vi "Drive Controller.vi"(8 "error in":errorcluster) -> ()   [LabVIEW 2017]
doc: "This VI executes continuously carrying out the current operation and responding to updates or new operation requests. It will often contain the timing or control code that is difficult to place directly in TeleOp. This VI generally opens all sensors and motors and isolates the rest of the robot code from knowing implementation details of how the operations are carried out."
uses:
  <vilib>/Rock Robotics/WPI/Framework/Completion Status.ctl
  Drive Setpoints.ctl
  Drive Operations.ctl
  Shared/RobotNeededPathData.ctl
  <vilib>/Rock Robotics/WPI/SafetyOutput/WPI_SafetyOutputConfigMenu.ctl
  <vilib>/Rock Robotics/SystemInterfaces/DIO/FPGA_DIOPWMChannel.ctl
  <vilib>/Rock Robotics/SystemInterfaces/DIO/FPGA_DIOChannel.ctl
  <vilib>/Rock Robotics/WPI/ThirdParty/Sensors/navX/_TypeDefs/FRIC_navX_DeviceNumbersTypeDef.ctl
  <vilib>/Rock Robotics/WPI/RobotDrive/WPI_RobotDriveOpen4MotorWithSPARK.vi
  <vilib>/Rock Robotics/WPI/Counter/WPI_CounterDigitalInputToDigitalSource.vi
  <vilib>/Rock Robotics/WPI/RobotDrive/WPI_RobotDriveOpen2MotorWithSPARK.vi
  <vilib>/addons/control/pid/pid.llb/PID (DBL).vi
  Drive Published Globals.vi
  <vilib>/addons/control/pid/NI_PID_pid.lvlib
  Configuration/Constants.vi
  Framework/Robot Global Data.vi
panel:
  in  "Integral Range":dbl=15.0
  out "PID Tuining":cluster{dbl, dbl}(graph)={170.0, 167.02}
  in  "Points":cluster{"X":dbl, "Y":dbl}[](array[cluster])=[{"X"=0.0, "Y"=0.0}, {"X"=0.01, "Y"=0.0}, {"X"=0.011, "Y"=0.17}, {"X"=1.0, "Y"=1.0}]
  in  "PID gains":T1={"proportional gain (Kc)"=0.01, "integral time (Ti, min)"=0.007, "derivative time (Td, min)"=0.0015} {"derivative time (Td, min)" format="%#_9g"}
  in  "Gains":T2={"FFV"=0.0059, "FFA"=0.0019, "Vel PID"={"P"=0.01, "I"=0.0, "D"=0.0}}
  in  "Interactive Values":T3={"Operation"=enum."Turn to Angle", "Left Speed"=-0.27, "Right Speed"=0.27, "Duration"=2.0, "Speed"=0.0, "Start Angle"=0.0, "Target Angle"=180.0, "Distance (inch)"=0.0, "Start Point (inch)"=0.0, "RobotNeededPathData"={"Path"=[], "MaxVel"=0.0, "MaxAccel"=-1.0, "Backwards?"=FALSE, "PointSpacing"=0.0, "LookaheadDist"=0.0, "Speed/Curve"=1.8, "SlowDistanceAtEnd"=12.0, "SlowSpeed"=15.0, "MaxDeAccel"=0.0}, "Start Point 2"=0.0} {"RobotNeededPathData"."SlowSpeed" format="%#_13g"; "RobotNeededPathData"."SlowDistanceAtEnd" format="%#_13g"; "RobotNeededPathData"."Speed/Curve" format="%#_13g"}
  in  "Buttons":cluster{"Execute Cmd":bool, "Abort Cmd":bool}
  out "Command Timing":cluster{"Start Time (ms)":u32, "Iterations":i32}={"Start Time (ms)"=372507, "Iterations"=0}
  out "Status":T6
  out "Setpoints":T7(graph)
  out "Current\nCmd":string="Started at  14:51:47.884\nDefault: Reserve,  L 0.0, R 0.0, D 0.000000"
  # "Tip: The graph shows the motor setpoints. It may also be helpful to observe inputs and sensor values.\nYou may also want to display tuning or debugging controls."
  # ".0088"
  # ".0017"
  # ".02"
  # "Interactive Command: You may fill in the settings for a command\nand schedule it with the Execute button. You can observe and abort\nany command while fine tuning the code for the controller."
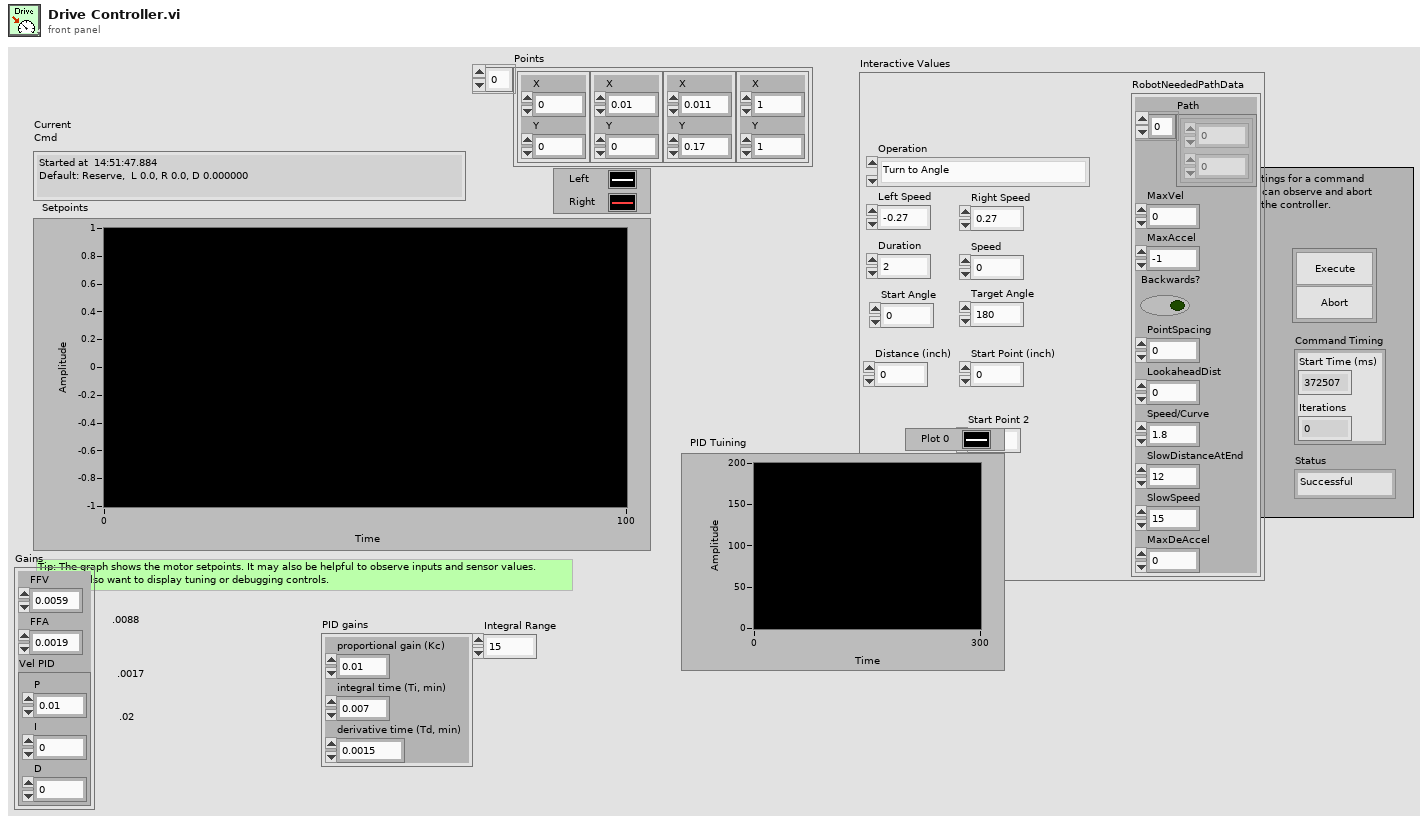
[diagram p1: front panel]
types:
  T1 = cluster{"proportional gain (Kc)":dbl, "integral time (Ti, min)":dbl, "derivative time (Td, min)":dbl}
  T2 = cluster{"FFV":dbl, "FFA":dbl, "Vel PID":cluster{"P":dbl, "I":dbl, "D":dbl}}
  T3 = typedef "Drive Setpoints.ctl" = cluster{"Operation":T4, "Left Speed":dbl, "Right Speed":dbl, "Duration":dbl, "Speed":dbl, "Start Angle":dbl, "Target Angle":dbl, "Distance (inch)":dbl, "Start Point (inch)":dbl, "RobotNeededPathData":T5, "Start Point 2":dbl}
  T4 = typedef "Drive Operations.ctl" = enum16{"Reserve", "Read Current", "Immediate", "Drive for Time", "Drive for Distance", "Turn to Angle", "Arc Turn", "Drive Path", "Drive To Cube"}
  T5 = typedef "RobotNeededPathData.ctl" = cluster{"Path":cluster{dbl, dbl}[], "MaxVel":dbl, "MaxAccel":dbl, "Backwards?":bool, "PointSpacing":dbl, "LookaheadDist":dbl, "Speed/Curve":dbl, "SlowDistanceAtEnd":dbl, "SlowSpeed":dbl, "MaxDeAccel":dbl}
  T6 = typedef "Completion Status.ctl" = enum16{"Successful", "Aborted", "Incomplete"}
  T7 = cluster{"Left Setpoint":dbl, "Right Setpoint":dbl}
  T8 = typedef "FPGA_DIOChannel.ctl" = enum8{"DIO 0", "DIO 1", "DIO 2", "DIO 3", "DIO 4", "DIO 5", "DIO 6", "DIO 7", "DIO 8", "DIO 9", "DIO MXP 0", "DIO MXP 1", "DIO MXP 2", "DIO MXP 3", "DIO MXP 4", "DIO MXP 5", "DIO MXP 6", "DIO MXP 7", "DIO MXP 8", "DIO MXP 9", "DIO MXP 10", "DIO MXP 11", "DIO MXP 12", "DIO MXP 13", "DIO MXP 14", "DIO MXP 15", "SPI Port CS1", "SPI Port CS2", "SPI Port CS3", "SPI Port MISO", "SPI Port MOSI", "Invalid"}
  T9 = typedef "FPGA_DIOPWMChannel.ctl" = enum8{"PWM 0", "PWM 1", "PWM 2", "PWM 3", "PWM 4", "PWM 5", "PWM 6", "PWM 7", "PWM 8", "PWM 9", "PWM MXP 0", "PWM MXP 1", "PWM MXP 2", "PWM MXP 3", "PWM MXP 4", "PWM MXP 5", "PWM MXP 6", "PWM MXP 7", "PWM MXP 8", "PWM MXP 9", "Invalid"}
  T10 = typedef "WPI_SafetyOutputConfigMenu.ctl" = enum16{"Enable", "Disable"}
  T11 = typedef "WPI_DigitalInputDevRef.ctl" = cluster{"DevStatus":errorcluster, "DIO Channel":T8}
  T12 = typedef "FPGA_CounterEncoderSourceConvertionLVSourceType.ctl" = cluster{"DevStatus":errorcluster, "AnalogTriggerMode?":bool, "DigitalMode":cluster{"DIO Channel":T13}, "AnalogTriggerMode":cluster{"AnalogTriggerIndex":T14, "OutputType":T15}}
  T13 = typedef "FPGA_DIODigitalSourceChannel.ctl" = enum8{"DIO 0", "DIO 1", "DIO 2", "DIO 3", "DIO 4", "DIO 5", "DIO 6", "DIO 7", "DIO 8", "DIO 9", "DIO MXP 0", "DIO MXP 1", "DIO MXP 2", "DIO MXP 3", "DIO MXP 4", "DIO MXP 5", "DIO MXP 6", "DIO MXP 7", "DIO MXP 8", "DIO MXP 9", "DIO MXP 10", "DIO MXP 11", "DIO MXP 12", "DIO MXP 13", "DIO MXP 14", "DIO MXP 15", "Disabled"}
  T14 = typedef "FPGA_AnalogTriggerIndex.ctl" = enum8{"Trig 0", "Trig 1", "Trig 2", "Trig 3", "Trig 4", "Trig 5", "Trig 6", "Trig 7", "Invalid"}
  T15 = typedef "FPGA_AnalogTriggerOutType.ctl" = enum16{"InWindow", "TriggerState", "Rising", "Falling"}
  T16 = typedef "WPI_RobotDriveDevRef.ctl" = cluster{"DevStatus":errorcluster, "Motors[]":T17[], "Square Inputs":bool, "Max Output":dbl}
  T17 = typedef "WPI_MotorControlDeviceRef.ctl" = cluster{"DeviceStatus":errorcluster, "Type":T18, "PWM":cluster{"PWM Channel":T9, "DeadBand":T19}, "CAN":cluster{"Device Number":u8, "SetOutput VI Ref":variant, "GetOutput VI Ref":variant, "Enable VI Ref":variant, "Disable VI Ref":variant, "Data":variant}, "Invert":bool, "DIO PWM":cluster{"PWM \"Enable\" Channel":T9, "DIOChannel":T8, "PWM Rate":dbl}}
  T18 = typedef "WPI_MotorControlType.ctl" = enum16{"PWM", "CAN", "DIO PWM"}
  T19 = typedef "WPI_PWMDeadband.ctl" = cluster{"Name":string, "maxPositivePwm":i32, "minPositivePwm":i32, "centerPwm":i32, "maxNegativePwm":i32, "minNegativePwm":i32, "angularRange":u16}
  T20 = typedef "WPI_EncoderDevRef.ctl" = cluster{"DevStatus":errorcluster, "EncoderIndex":T21, "CounterIndex":T22, "DistancePerCount":dbl, "Decoding Type":T23}
  T21 = typedef "FPGA_EncoderIdx.ctl" = enum8{"Enc 0", "Enc 1", "Enc 2", "Enc 3", "Enc 4", "Enc 5", "Enc 6", "Enc 7", "Invalid"}
  T22 = typedef "FPGA_CounterCtrSystemIndex.ctl" = enum8{"Ctr 0", "Ctr 1", "Ctr 2", "Ctr 3", "Ctr 4", "Ctr 5", "Ctr 6", "Ctr 7", "Invalid"}
  T23 = typedef "WPI_EncoderType.ctl" = enum16{"1x", "2x", "4x"}
  T24 = typedef "Command Status Info.ctl" = cluster{"Name":string, "Status":T6, "notifier out":T25}
  T25 = typedef "Completion Notifier.ctl" = refnum<notifier>
  T26 = cluster{"SubSystem Data":T3, cluster{"Start Time (ms)":u32, "Iterations":i32}, cluster{"Command Info":T24, "Description":string, "Default Command":T3, "queue out":refnum<queue>, "Subsystem Name":string}}
  T27 = typedef "FRIC_navX_DeviceNumbersTypeDef.ctl" = enum16{"Dev0", "Dev1", "Dev2", "Dev3"}
  T28 = cluster{"dx/dt":dbl, "dx/dt":dbl, "Yaw":dbl, cluster{dbl, dbl}}
  T29 = cluster{"LeftDistance":dbl, "RightDistance":dbl, "LeftVelocity":dbl, "RightVelocity":dbl, "Angle":dbl, "Location":cluster{dbl, dbl}}
  T30 = cluster{"Yaw":dbl, "Roll":dbl, "Pitch":dbl, "Heading":dbl, "Fused Heading":dbl}
  T31 = cluster{"SubSystem Data":T3, cluster{"Start Time (ms)":u32, "Iterations":i32}, "Default Command Arguments":cluster{"Command Info":T24, "Description":string, "Default Command":T3, "queue out":refnum<queue>, "Subsystem Name":string}}
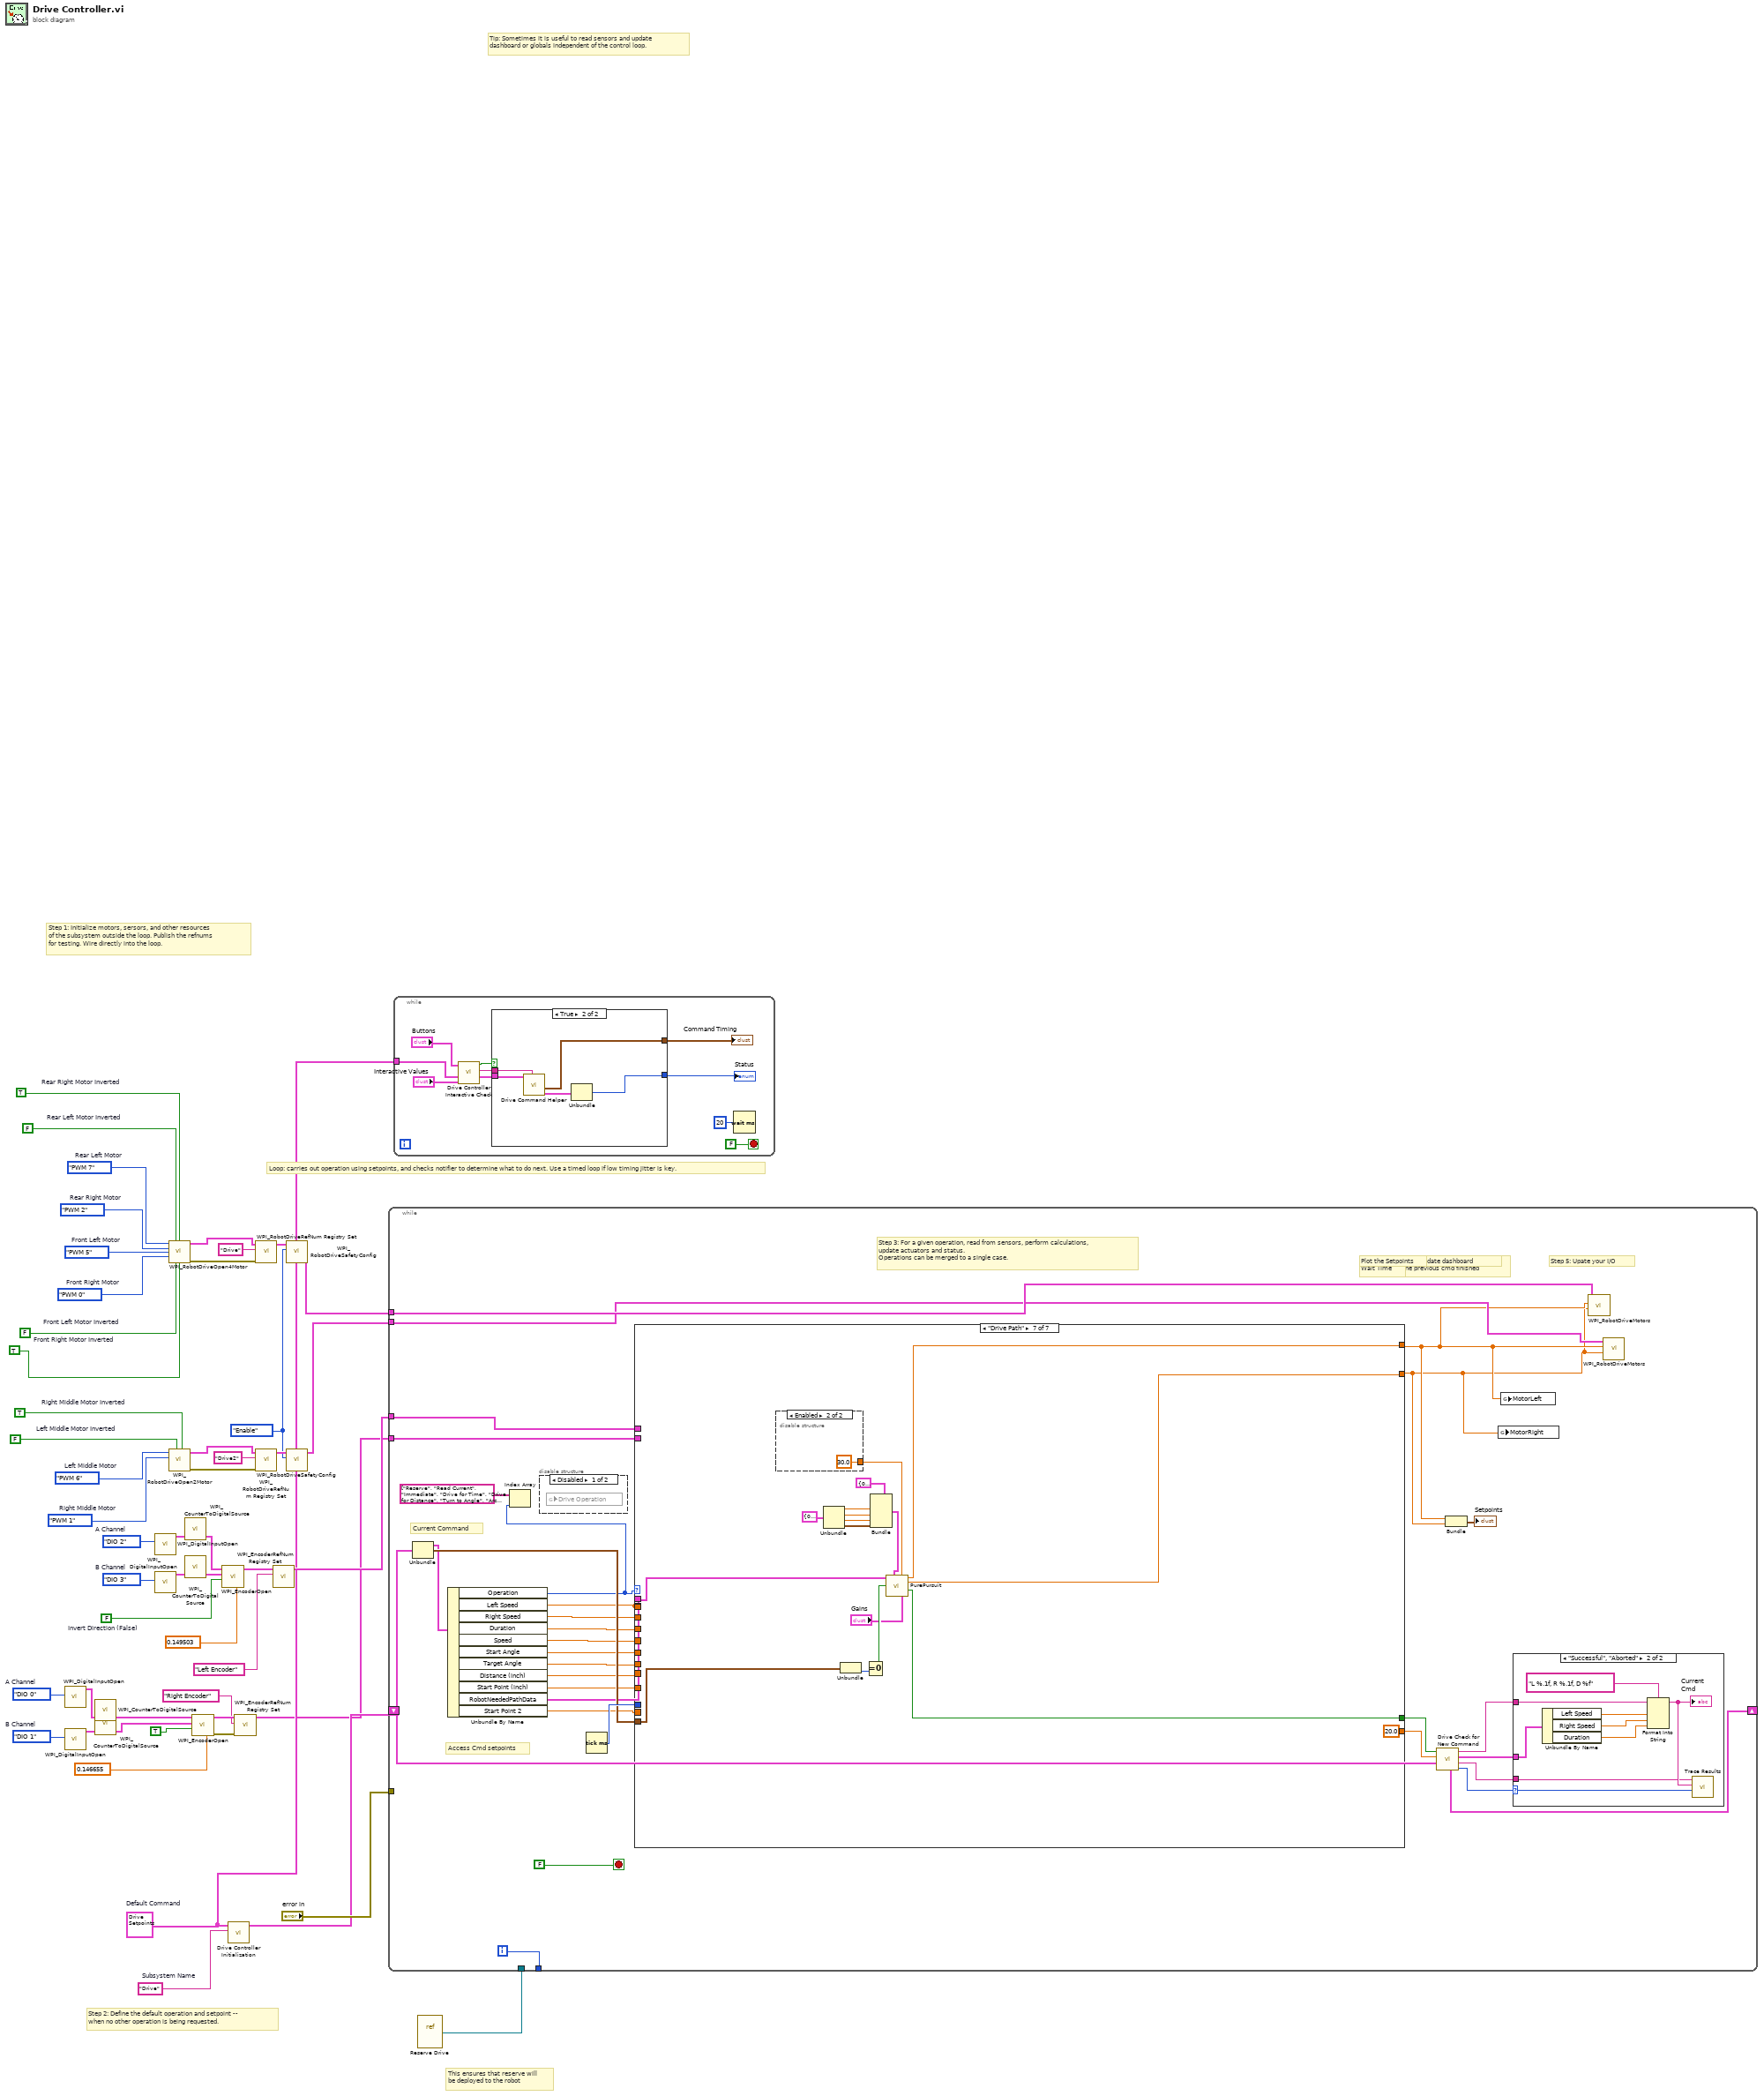
[diagram p0: block diagram]
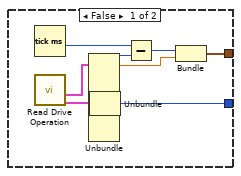
[diagram p2: hidden frame]
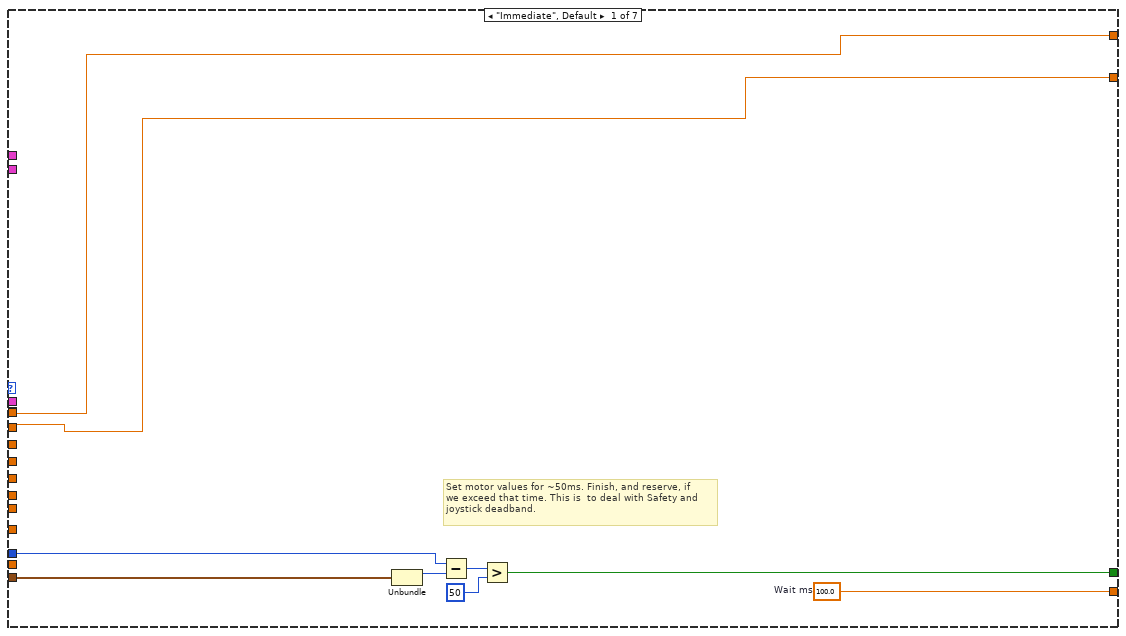
[diagram p4: hidden frame]
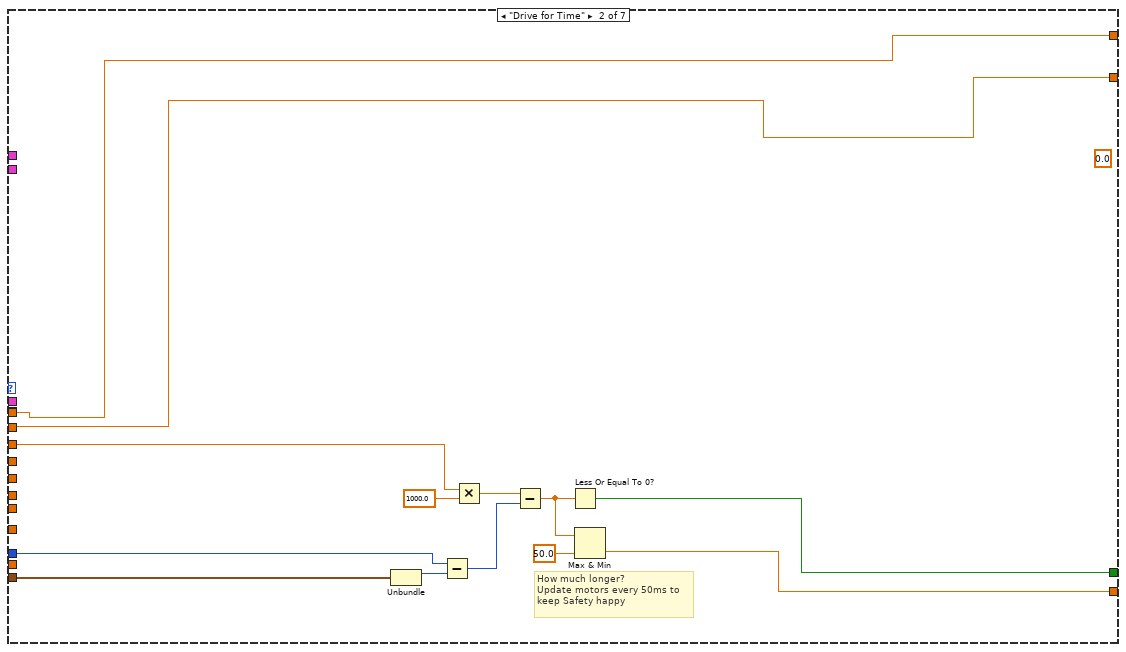
[diagram p5: hidden frame]
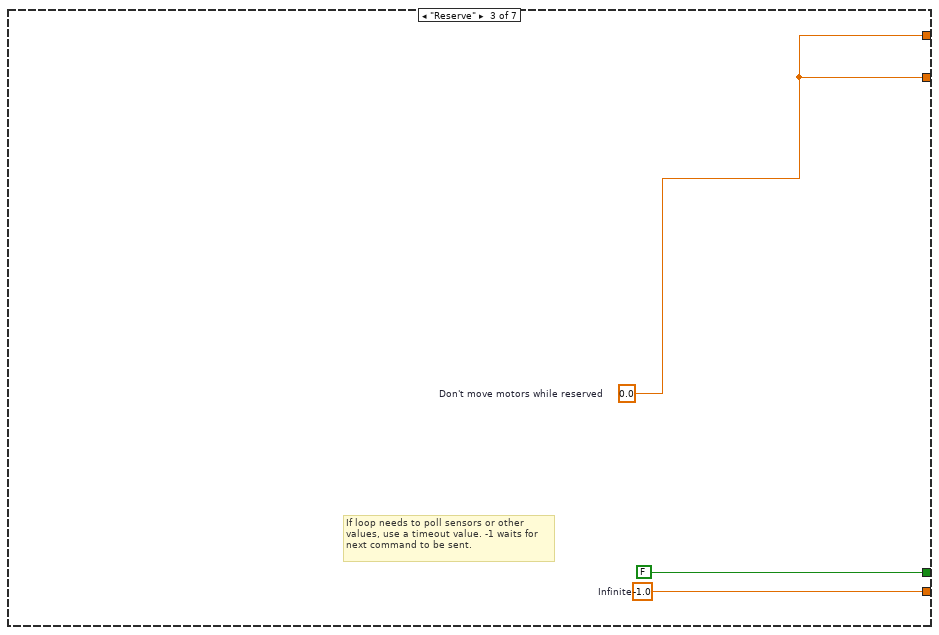
[diagram p6: hidden frame]
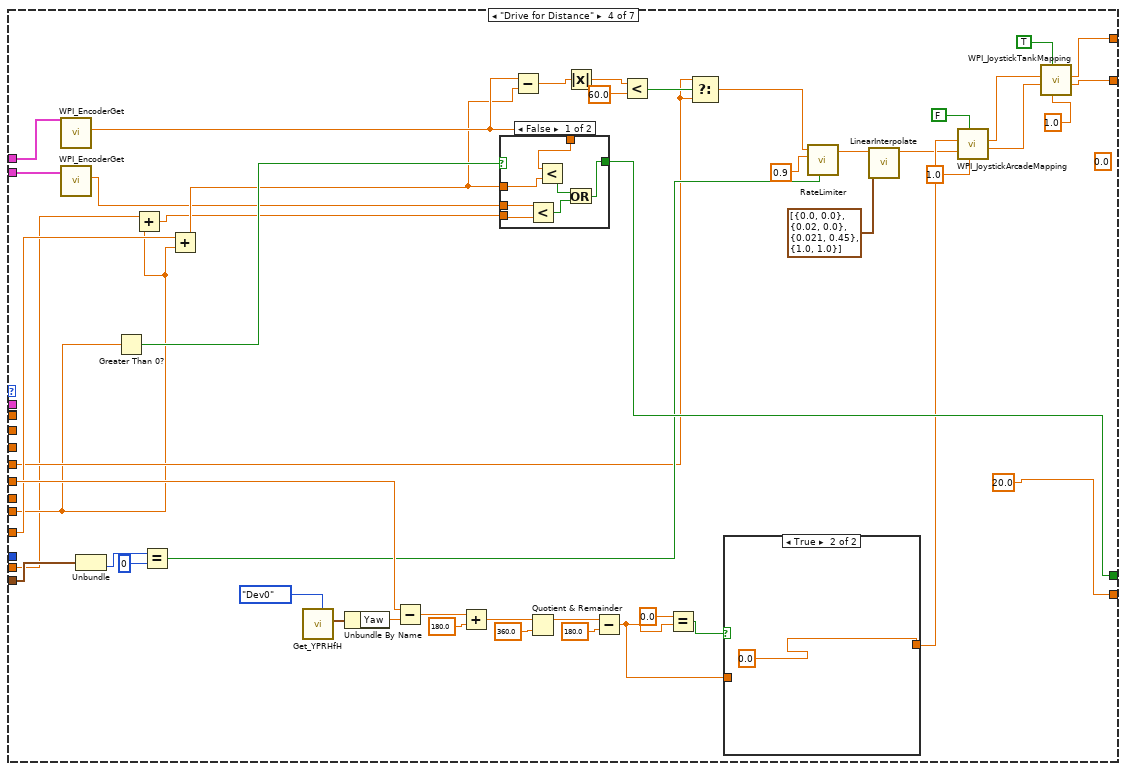
[diagram p7: hidden frame]
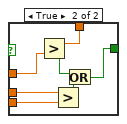
[diagram p8: hidden frame]
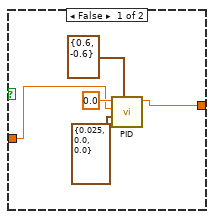
[diagram p9: hidden frame]
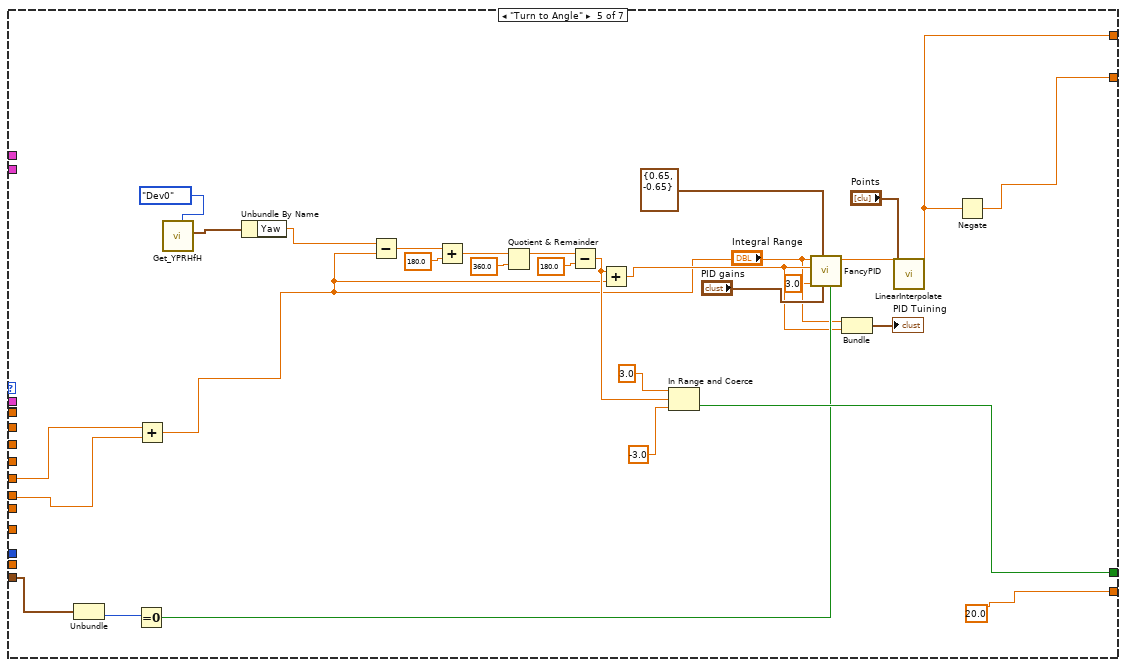
[diagram p10: hidden frame]
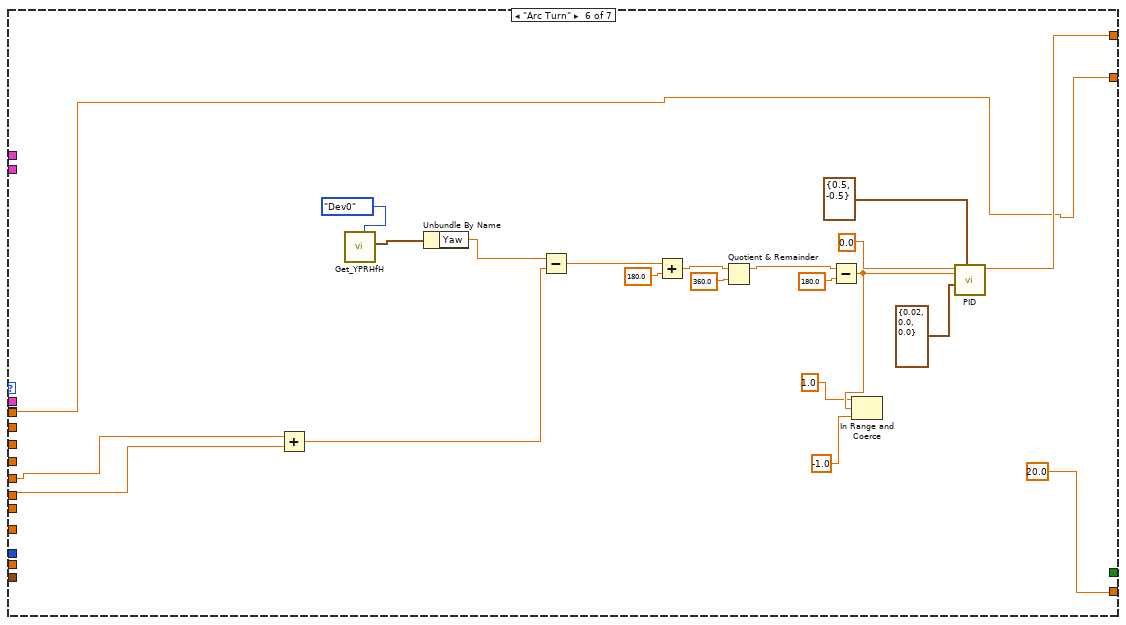
[diagram p11: hidden frame]
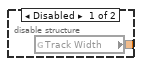
[diagram p12: hidden frame]
diagram:
  w4 = FPGA_DIOChannel."DIO 1"  # B Channel
  w7 = FPGA_DIOChannel."DIO 0"  # A Channel
  w13 = T3 {"Operation"=enum."Reserve", "Left Speed"=0.0, "Right Speed"=0.0, "Duration"=0.0, "Speed"=0.0, "Start Angle"=0.0, "Target Angle"=0.0, "Distance (inch)"=0.0, "Start Point (inch)"=0.0, "RobotNeededPathData"={"Path"=[], "MaxVel"=0.0, "MaxAccel"=0.0, "Backwards?"=FALSE, "PointSpacing"=0.0, "LookaheadDist"=0.0, "Speed/Curve"=1.8, "SlowDistanceAtEnd"=12.0, "SlowSpeed"=15.0, "MaxDeAccel"=0.0}, "Start Point 2"=0.0}  # Default Command
  w20 = TRUE  # Right Middle Motor Inverted
  w21 = FALSE  # Left Middle Motor Inverted
  w24 = FPGA_DIOPWMChannel."PWM 1"  # Right Middle Motor
  w25 = FPGA_DIOPWMChannel."PWM 6"  # Left Middle Motor
  w34 = FALSE  # Invert Direction (False)
  w27 = FPGA_DIOChannel."DIO 3"  # B Channel
  w28 = FPGA_DIOChannel."DIO 2"  # A Channel
  w36 = TRUE  # Front Right Motor Inverted
  w37 = FALSE  # Front Left Motor Inverted
  w38 = TRUE  # Rear Right Motor Inverted
  w39 = FALSE  # Rear Left Motor Inverted
  w40 = FPGA_DIOPWMChannel."PWM 0"  # Front Right Motor
  w41 = FPGA_DIOPWMChannel."PWM 5"  # Front Left Motor
  w42 = FPGA_DIOPWMChannel."PWM 2"  # Rear Right Motor
  w43 = FPGA_DIOPWMChannel."PWM 7"  # Rear Left Motor
  w15 = WPI_SafetyOutputConfigMenu."Enable" ("mode")
  w51 = "Drive"  # Subsystem Name
  # "Step 1: Initialize motors, sersors, and other resources\nof the subsystem outside the loop. Publish the refnums\nfor testing. Wire directly into the loop."
  # "Step 2: Define the default operation and setpoint --\nwhen no other operation is being requested."
  # "This ensures that reserve will\nbe deployed to the robot"
  # "Tip: Sometimes it is useful to read sensors and update\ndashboard or globals independent of the control loop."
  # "Loop: carries out operation using setpoints, and checks notifier to determine what to do next. Use a timed loop if low timing jitter is key."
  n1 = call <vilib>:"WPI_DigitalInputOpen.vi"("DIO Channel"=w7) -> ("DigitalInputDevRef"=w8:T11)  [unwired: 1 in, 9 out]
  n2 = call <vilib>:"WPI_DigitalInputOpen.vi"("DIO Channel"=w4) -> ("DigitalInputDevRef"=w5:T11)  [unwired: 1 in, 9 out]
  n3 = call-poly <vilib>:"WPI_CounterToDigitalSource.vi"("DigitalInputDevRef"=w8) -> ("Digital Source"=w9:T12)  [unwired: 6 out]
  n4 = call-poly <vilib>:"WPI_CounterToDigitalSource.vi"("DigitalInputDevRef"=w5) -> ("Digital Source"=w6:T12)  [unwired: 6 out]
  n5 = call <vilib>:"WPI_DigitalInputOpen.vi"("DIO Channel"=w28) -> ("DigitalInputDevRef"=w31:T11)  [unwired: 1 in, 9 out]
  n6 = call <vilib>:"WPI_DigitalInputOpen.vi"("DIO Channel"=w27) -> ("DigitalInputDevRef"=w30:T11)  [unwired: 1 in, 9 out]
  n7 = call-poly <vilib>:"WPI_RobotDriveOpen4Motor.vi"("Rear Left Motor"=w43, "Rear Left Motor Inverted"=w39, "Rear Right Motor Inverted"=w38, "Rear Right Motor"=w42, "Front Left Motor"=w41, "Front Right Motor"=w40, "Front Left Motor Inverted"=w37, "Front Right Motor Inverted"=w36) -> ("RobotDriveDevRef"=w50:T16, "error out"=w48:errorcluster)  [unwired: 6 in]
  n8 = call-poly <vilib>:"WPI_RobotDriveOpen2Motor.vi"("Right Motor Inverted"=w20, "Left Motor Inverted"=w21, "Right Motor"=w24, "Left Motor"=w25) -> ("error out"=w19:errorcluster, "RobotDriveDevRef"=w23:T16)  [unwired: 6 in]
  n9 = call-poly <vilib>:"WPI_CounterToDigitalSource.vi"("DigitalInputDevRef"=w31) -> ("Digital Source"=w32:T12)  [unwired: 6 out]
  n10 = call-poly <vilib>:"WPI_CounterToDigitalSource.vi"("DigitalInputDevRef"=w30) -> ("Digital Source"=w29:T12)  [unwired: 6 out]
  n11 = call <vilib>:"WPI_EncoderOpen.vi"("DistancePerCount"=0.146655, "Invert Direction (False)"=TRUE, "BSource"=w6, "ASource"=w9) -> ("error out"=w11:errorcluster, "EncoderDevRef"=w10:T20)  [unwired: 4 in, 2 out]
  n12 = call <vilib>:"WPI_EncoderOpen.vi"("DistancePerCount"=0.149503, "Invert Direction (False)"=w34, "BSource"=w29, "ASource"=w32) -> ("EncoderDevRef"=w33:T20)  [unwired: 4 in, 3 out]
  n13 = call "Drive Controller Initialization.vi"("Subsystem Name"=w51, "Default Command"=w13) -> ("Current Command"=w45:T26)  [unwired: 9 in]
  n14 = call <vilib>:"WPI_EncoderRefNum Registry Set.vi"("error in (no error)"=w11, "refnum name"="Right Encoder", "EncoderDevRef"=w10) -> ("EncoderDevRef"=w12:T20)  [unwired: 7 in, 1 out]
  n15 = call <vilib>:"WPI_RobotDriveRefNum Registry Set.vi"("error in (no error)"=w48, "refnum name"="Drive", "RobotDriveDevRef"=w50) -> ("RobotDriveDevRef"=w18:T16)  [unwired: 1 in, 7 out]
  n16 = call <vilib>:"WPI_RobotDriveRefNum Registry Set.vi"("error in (no error)"=w19, "refnum name"="Drive2", "RobotDriveDevRef"=w23) -> ("RobotDriveDevRef"=w17:T16)  [unwired: 7 in, 1 out]
  n17 = call <vilib>:"WPI_EncoderRefNum Registry Set.vi"("refnum name"="Left Encoder", "EncoderDevRef"=w33) -> ("EncoderDevRef"=w26:T20)  [unwired: 8 in, 1 out]
  n18 = call <vilib>:"WPI_RobotDriveSafetyConfig.vi"("mode"=w15, "RobotDriveDevRef"=w18) -> ("RobotDriveDevRef"=w47:T16)  [unwired: 8 in, 1 out]
  n19 = call <vilib>:"WPI_RobotDriveSafetyConfig.vi"("mode"=w15, "RobotDriveDevRef"=w17) -> ("RobotDriveDevRef"=w16:T16)  [unwired: 8 in, 1 out]
  n20 = while {
    tunnel: w13 -> [w53]
    stop <- FALSE stop-if-true
    n21 = call "Drive Controller Interactive Check.vi"("Interactive Command In"="Interactive Values", "Default Command"=w53, "Buttons"="Buttons") -> ("Interactive Command Out"=w55:T3, "Trace String"=w56:string, "Schedule"=w57:bool)  [unwired: 6 in]
    n22 = case shown="True" w57 {
      tunnel: [w66 w74] -> w58
      tunnel: [w65 w70] -> w59
      tunnel: w56 -> [_ w72]
      tunnel: w55 -> [_ w71]
      frame False {
        n23 = Tick Count (ms)() -> (millisecond timer value=w69:u32)
        n24 = call "Read Drive Operation.vi"() -> ("Command Info"=w63:T24, "SubSystem Data"=w62:T3)  [unwired: 9 in, 1 out]
        n25 = Unbundle(w62) -> ("Operation"=w67:T4, "Left Speed"=w64:dbl)  [unwired: 9 out]
        n26 = Unbundle(w63) -> ("Status"=w66:T6)  [unwired: 2 out]
        n27 = Subtract(x=w69, y=w67) -> (x-y=w68:u32)
        n28 = Bundle(w68, "Left Speed"=w64) -> (w65:cluster{u32, "Left Speed":dbl})  [unwired: 1 in]
      }
      frame True {
        n29 = call "Drive Command Helper.vi"("Description"=w72, "SubSystem Data"=w71) -> ("Command Info Out"=w73:T24, "Command Timing"=w70:cluster{"Start Time (ms)":u32, "Iterations":i32})  [unwired: 7 in, 1 out]
        n30 = Unbundle(w73) -> ("Status"=w74:T6)  [unwired: 2 out]
      }
    }
    "Status" <- w58
    "Command Timing" <- w59
    n31 = Wait (ms)(milliseconds to wait=u32 20) -> ()  [unwired: 1 out]
  }
  n32 = vi-ref "Reserve Drive.vi"() -> (w44:refnum<vi>)
  n33 = while {
    shift-right: [w102] -> _
    shift-left: w45 -> [w75]
    tunnel: [w105] -> _
    tunnel: w47 -> [w84]
    tunnel: "error in" -> [_]
    tunnel: w44 -> [_]
    tunnel: w26 -> [w82]
    tunnel: w16 -> [w83]
    tunnel: w12 -> [w81]
    i -> [w105]
    stop <- FALSE stop-if-true
    # "Plot the Setpoints"
    # "Step 5: Upate your I/O"
    # "Step 4: Format a string to describe this\ncmd and how the previous cmd finished"
    # "Current Command"
    # "Update motors and update dashboard"
    # "Access Cmd setpoints"
    # "Finished? &\nWait Time"
    # "Step 3: For a given operation, read from sensors, perform calculations,\nupdate actuators and status.\nOperations can be merged to a single case."
    n34 = Unbundle(w75) -> ("SubSystem Data"=w85:T3, w96:cluster{"Start Time (ms)":u32, "Iterations":i32})  [unwired: 1 out]
    n35 = Unbundle By Name(w85) -> ("Operation"=w77:T4, "Left Speed"=w94:dbl, "Right Speed"=w93:dbl, "Duration"=w92:dbl, "Speed"=w91:dbl, "Start Angle"=w90:dbl, "Target Angle"=w89:dbl, "Distance (inch)"=w88:dbl, "Start Point (inch)"=w87:dbl, "RobotNeededPathData"=w86:T5, "Start Point 2"=w80:dbl)
    n36 = Index Array(array=string[] ["Reserve", "Read Current", "Immediate", "Drive for Time", "Drive for Distance", "Turn to Angle", "Arc Turn", "Drive Path", "Drive To Cube"] ("Strings []"), index=w77) -> ()  [unwired: 1 out]
    n37 = disable-structure shown="Disabled" {
      frame Disabled {
        n38 = global read "Robot Global Data.vi" "Drive Operation"() -> ()  [unwired: 1 in]
      }
      frame Enabled {
      }
    }
    n39 = Tick Count (ms)() -> (millisecond timer value=w104:u32)
    n40 = case shown="\"Drive Path\"" w77 {
      tunnel: [w115 w119 w131 20.0 ("Infinite") 20.0 ("Infinite") 20.0 ("Infinite") 20.0 ("Infinite")] -> w101
      tunnel: [w110 w123 FALSE ("ignore previous (F)") w167 w222 _ w264] -> w100
      tunnel: w96 -> [w109 w125 _ w148 w212 _ w263]
      tunnel: w104 -> [w111 w122 _ _ _ _ _]
      tunnel: [w108 w117 w129 w153 w210 w231 w266] -> w79
      tunnel: [w107 w116 w129 w154 w209 w230 w265] -> w78
      tunnel: w91 -> [_ _ _ w137 _ _ _]
      tunnel: w88 -> [_ _ _ w135 _ _ _]
      tunnel: w92 -> [_ w118 _ _ _ _ _]
      tunnel: w94 -> [w108 _ _ _ _ w230 _]
      tunnel: w93 -> [w107 w116 _ _ _ _ _]
      tunnel: w82 -> [_ _ _ w165 _ _ _]
      tunnel: w90 -> [_ _ _ w161 w225 w234 _]
      tunnel: w89 -> [_ _ _ _ w224 w233 _]
      tunnel: w87 -> [_ _ _ w160 _ _ _]
      tunnel: w94 -> [_ w117 _ _ _ _ _]
      tunnel: w86 -> [_ _ _ _ _ _ w267]
      tunnel: w81 -> [_ _ _ w136 _ _ _]
      tunnel: w80 -> [_ _ _ w134 _ _ _]
      frame "Immediate", Default {
        w115 = 100.0  # Wait ms
        # "Set motor values for ~50ms. Finish, and reserve, if\nwe exceed that time. This is  to deal with Safety and\njoystick deadband."
        n41 = Unbundle(w109) -> ("Start Time (ms)"=w112:u32)  [unwired: 1 out]
        n42 = Subtract(x=w111, y=w112) -> (x-y=w113:u32)
        n43 = Greater?(x=w113, y=u8 50 ("Left Motor")) -> (0:w110:bool)
      }
      frame "Drive for Time" {
        (unwired) 0.0 ("output")
        # "How much longer?\nUpdate motors every 50ms to\nkeep Safety happy"
        n44 = Unbundle(w125) -> ("Start Time (ms)"=w124:u32)  [unwired: 1 out]
        n45 = Subtract(x=w122, y=w124) -> (x-y=w128:u32)
        n46 = Multiply(x=w118, y=1000.0) -> (x*y=w127:dbl)
        n47 = Subtract(x=w127, y=w128) -> (x-y=w121:dbl)
        n48 = Less Or Equal To 0?(x=w121) -> (x <= 0?=w123:bool)
        n49 = Max & Min(x=w121, y=50.0) -> (min(x,y)=w119:dbl)  [unwired: 1 out]
      }
      frame "Reserve" {
        w129 = 0.0  # Don't move motors while reserved
        w131 = -1.0  # Infinite
        # "If loop needs to poll sensors or other\nvalues, use a timeout value. -1 waits for\nnext command to be sent."
      }
      frame "Drive for Distance" {
        (unwired) 0.0 ("output")
        n50 = call <vilib>:"WPI_EncoderGet.vi"("EncoderDevRef"=w165) -> ("Distance"=w144:dbl)  [unwired: 5 in, 5 out]
        n51 = call <vilib>:"WPI_EncoderGet.vi"("EncoderDevRef"=w136) -> ("Distance"=w132:dbl)  [unwired: 5 in, 5 out]
        n52 = Unbundle(w148) -> ("Iterations"=w147:i32)  [unwired: 1 out]
        n53 = Greater Than 0?(x=w135) -> (x > 0?=w159:bool)
        n54 = Add(x=w134, y=w135) -> (x+y=w133:dbl)
        n55 = Equal?(x=w147, y=0) -> (x = y?=w145:bool)
        n56 = Add(x=w160, y=w135) -> (x+y=w143:dbl)
        n57 = call <vilib>:"Get_YPRHfH.vi"("Device Number"=FRIC_navX_DeviceNumbersTypeDef."Dev0") -> ("YRPHfH"=w179:T30)  [unwired: 10 in]
        n58 = Unbundle By Name(w179) -> ("Yaw"=w170:dbl)
        n59 = Subtract(x=w161, y=w170) -> (x-y=w169:dbl)
        n60 = Add(x=w169, y=180.0) -> (x+y=w174:dbl)
        n61 = case shown="False" w159 {
          tunnel: w144 -> [w185 w193]
          tunnel: w143 -> [w186 w192]
          tunnel: [w183 w187] -> w167
          tunnel: w133 -> [w181 w191]
          tunnel: w132 -> [w182 w190]
          frame False {
            n62 = Less?(x=w182, y=w181) -> (x < y?=w180:bool)
            n63 = Less?(x=w185, y=w186) -> (x < y?=w184:bool)
            n64 = Or(x=w184, y=w180) -> (x .or. y?=w183:bool)
          }
          frame True {
            n65 = Greater?(x=w193, y=w192) -> (0:w189:bool)
            n66 = Greater?(x=w190, y=w191) -> (0:w188:bool)
            n67 = Or(x=w189, y=w188) -> (x .or. y?=w187:bool)
          }
        }
        n68 = Subtract(x=w144, y=w143) -> (x-y=w142:dbl)
        n69 = Quotient & Remainder(x=w174, y=360.0) -> (x-y*floor(x/y)=w172:dbl)  [unwired: 1 out]
        n70 = Absolute Value(x=w142) -> (abs(x)=w141:dbl)
        n71 = Subtract(x=w172, y=180.0) -> (x-y=w168:dbl)
        n72 = Less?(x=w141, y=60.0) -> (x < y?=w139:bool)
        n73 = Equal?(x=0.0, y=w168) -> (x = y?=w177:bool)
        n74 = Select(t=w137, s=w139, f=w137) -> (s? t:f=w138:dbl)
        n75 = case shown="True" w177 {
          tunnel: [w194 0.0] -> w162
          tunnel: w168 -> [w195 _]
          frame False {
            n76 = call-poly <vilib>:"PID.vi"("output range"=cluster{"output high":dbl, "output low":dbl} {"output high"=0.6, "output low"=-0.6}, "PID gains"=T1 {"proportional gain (Kc)"=0.025, "integral time (Ti, min)"=0.0, "derivative time (Td, min)"=0.0}, "process variable"=w195, "setpoint"=0.0) -> ("output"=w194:dbl)  [unwired: 6 in, 1 out]
          }
          frame True {
          }
        }
        n77 = call "RateLimiter.vi"("Reset"=w145, "Max dx/dt"=0.9, "Input"=w138) -> ("Output"=w156:dbl)  [unwired: 8 in]
        n78 = call "LinearInterpolate.vi"("Points"=cluster{"X":dbl, "Y":dbl}[] [{"X"=0.0, "Y"=0.0}, {"X"=0.02, "Y"=0.0}, {"X"=0.021, "Y"=0.45}, {"X"=1.0, "Y"=1.0}], "Value"=w156) -> ("Output"=w157:dbl)  [unwired: 9 in]
        n79 = call <vilib>:"WPI_JoystickArcadeMapping.vi"("Max Output"=1.0, "Square Inputs"=FALSE, "Y axis value"=w157, "X axis value"=w162) -> ("Right Motor Value"=w152:dbl, "Left Motor Value"=w151:dbl)  [unwired: 6 in]
        n80 = call <vilib>:"WPI_JoystickTankMapping.vi"("Max Output"=1.0, "Square Inputs"=TRUE, "Right axis value"=w152, "Left axis value"=w151) -> ("Right Motor Value"=w154:dbl, "Left Motor Value"=w153:dbl)  [unwired: 6 in]
      }
      frame "Turn to Angle" {
        n81 = Unbundle(w212) -> ("Iterations"=w211:i32)  [unwired: 1 out]
        n82 = Equal To 0?(x=w211) -> (x = 0?=w205:bool)
        n83 = Add(x=w225, y=w224) -> (x+y=w202:dbl)
        n84 = call <vilib>:"Get_YPRHfH.vi"("Device Number"=FRIC_navX_DeviceNumbersTypeDef."Dev0") -> ("YRPHfH"=w227:T30)  [unwired: 10 in]
        n85 = Unbundle By Name(w227) -> ("Yaw"=w215:dbl)
        n86 = Subtract(x=w215, y=w202) -> (x-y=w216:dbl)
        n87 = Add(x=w216, y=180.0) -> (x+y=w219:dbl)
        n88 = Quotient & Remainder(x=w219, y=360.0) -> (x-y*floor(x/y)=w217:dbl)  [unwired: 1 out]
        n89 = Subtract(x=w217, y=180.0) -> (x-y=w214:dbl)
        n90 = Add(x=w214, y=w202) -> (x+y=w203:dbl)
        n91 = In Range and Coerce(upper limit=3.0, x=w214, lower limit=-3.0) -> (In Range?=w222:bool)  [unwired: 1 out]
        n92 = call "FancyPID.vi"("Reset"=w205, "Gains"="PID gains", "Range"=cluster{"output high":dbl, "output low":dbl} {"output high"=0.65, "output low"=-0.65} ("output range"), "Disable Range"=3.0, "Integral Range"="Integral Range", "Process variable"=w203, "Setpoint"=w202) -> ("output"=w206:dbl)  [unwired: 4 in]
        n93 = Bundle(w202, w203) -> (→"PID Tuining":cluster{dbl, dbl})  [unwired: 1 in]
        n94 = call "LinearInterpolate.vi"("Points"="Points", "Value"=w206) -> ("Output"=w210:dbl)  [unwired: 9 in]
        n95 = Negate(x=w210) -> (-x=w209:dbl)
      }
      frame "Arc Turn" {
        n96 = Add(x=w234, y=w233) -> (x+y=w241:dbl)
        n97 = call <vilib>:"Get_YPRHfH.vi"("Device Number"=FRIC_navX_DeviceNumbersTypeDef."Dev0") -> ("YRPHfH"=w237:T30)  [unwired: 10 in]
        n98 = Unbundle By Name(w237) -> ("Yaw"=w235:dbl)
        n99 = Subtract(x=w235, y=w241) -> (x-y=w243:dbl)
        n100 = Add(x=w243, y=180.0) -> (x+y=w246:dbl)
        n101 = Quotient & Remainder(x=w246, y=360.0) -> (x-y*floor(x/y)=w244:dbl)  [unwired: 1 out]
        n102 = Subtract(x=w244, y=180.0) -> (x-y=w240:dbl)
        n103 = In Range and Coerce(upper limit=1.0, x=w240, lower limit=-1.0) -> ()  [unwired: 2 out]
        n104 = call-poly <vilib>:"PID.vi"("output range"=cluster{"output high":dbl, "output low":dbl} {"output high"=0.5, "output low"=-0.5}, "PID gains"=T1 {"proportional gain (Kc)"=0.02, "integral time (Ti, min)"=0.0, "derivative time (Td, min)"=0.0}, "process variable"=w240, "setpoint"=0.0) -> ("output"=w231:dbl)  [unwired: 6 in, 1 out]
      }
      frame "Drive Path" {
        n105 = disable-structure shown="Enabled" {
          disable-tunnel: [w268 30.0 ("Trackwidth")] -> w253
          frame Disabled {
            n106 = global read "Constants.vi" "Track Width"() -> (w268:dbl)
          }
          frame Enabled {
          }
        }
        n107 = Unbundle(T28 {"dx/dt"=0.0, "dx/dt"=0.0, "Yaw"=0.0, {0.0, 0.0}} ("cluster")) -> ("dx/dt"=w260:dbl, "dx/dt"=w259:dbl, "Yaw"=w258:dbl, w257:cluster{dbl, dbl})
        n108 = Unbundle(w263) -> ("Iterations"=w254:i32)  [unwired: 1 out]
        n109 = Equal To 0?(x=w254) -> (x = 0?=w255:bool)
        n110 = Bundle(cluster=T29 {"LeftDistance"=0.0, "RightDistance"=0.0, "LeftVelocity"=0.0, "RightVelocity"=0.0, "Angle"=0.0, "Location"={0.0, 0.0}} ("SensorData"), "LeftVelocity"=w260, "RightVelocity"=w259, "Angle"=w258, "Location"=w257) -> (w261:T29)  [unwired: 2 in]
        n111 = call "PurePursuit.vi"("RobotNeededPathData"=w267, "SensorData"=w261, "Trackwidth"=w253, "Reset"=w255, "Gains"="Gains") -> ("LeftValue"=w266:dbl, "RightValue"=w265:dbl, "Done"=w264:bool)  [unwired: 6 in, 2 out]
      }
    }
    n112 = call "Drive Check for New Command.vi"("input cluster"=w75, "Wait time (ms)"=w101, "Finished?"=w100) -> ("Completion"=w103:T6, "Subsystem Name"=w97:string, "Current Command"=w98:T3, "Initial Trace String"=w99:string, "Next Command"=w102:T31)  [unwired: 4 in]
    n113 = Bundle("LeftValue"=w79, "RightValue"=w78) -> (→"Setpoints":cluster{"LeftValue":dbl, "RightValue":dbl})  [unwired: 1 in]
    n114 = global write "Drive Published Globals.vi" "MotorRight"(w78) -> ()
    n115 = global write "Drive Published Globals.vi" "MotorLeft"(w79) -> ()
    n116 = case shown="\"Successful\", \"Aborted\"" w103 {
      selector: w103 -> [_ w278]
      tunnel: w99 -> [_ w273]
      tunnel: w98 -> [_ w274]
      tunnel: w97 -> [_ w270]
      frame "Incomplete", Default {
        # "Continuing current command"
      }
      frame "Successful", "Aborted" {
        # "Report and setup for next command"
        n117 = Unbundle By Name(w274) -> ("Left Speed"=w276:dbl, "Right Speed"=w277:dbl, "Duration"=w271:dbl)
        n118 = Format Into String(format string="L %.1f, R %.1f, D %f", initial string=w273, w276, w277, w271) -> (resulting string=w272:string)  [unwired: 1 in, 1 out]
        "Current\nCmd" <- w272
        n119 = call <vilib>:"Trace Results.vi"("Status of previous command"=w278, "Description"=w272, "Subsystem"=w270) -> ()  [unwired: 9 in]
      }
    }
    n120 = call <vilib>:"WPI_RobotDriveMotors.vi"("RightSpeed"=w78, "LeftSpeed"=w79, "RobotDriveDevRef"=w84) -> ()  [unwired: 1 in, 8 out]
    n121 = call <vilib>:"WPI_RobotDriveMotors.vi"("RightSpeed"=w78, "LeftSpeed"=w79, "RobotDriveDevRef"=w83) -> ()  [unwired: 1 in, 8 out]
  }
